vi "three string pad with zeroes.vi"(3 "String 3 input":string, 4 "String 2 input":string, 5 "String 1 input":string) -> (0 "String 3 output":string, 1 "String 2 output":string, 2 "String 1 output":string)   [LabVIEW 2017]
doc: "This takes two strings (presumably of 0s and 1s), and pads the shorter one with zeroes so that it has the same length as the longer one."
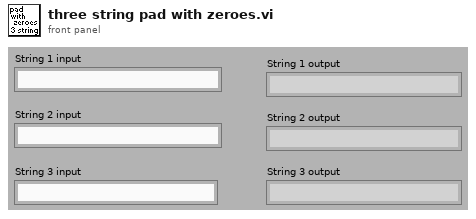
[diagram p1: front panel]
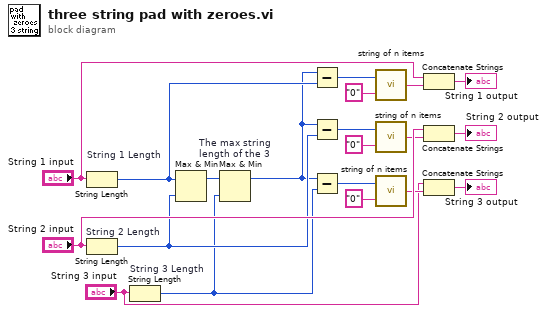
[diagram p0: block diagram]
diagram:
  n1 = String Length "String 1 Length"(string="String 1 input") -> (length=w9:i32)
  n2 = String Length "String 2 Length"(string="String 2 input") -> (length=w10:i32)
  n3 = String Length "String 3 Length"(string="String 3 input") -> (length=w1:i32)
  n4 = Max & Min(x=w9, y=w10) -> (max(x,y)=w8:i32)  [unwired: 1 out]
  n5 = Max & Min "The max string \nlength of the 3"(x=w8, y=w1) -> (max(x,y)=w2:i32)  [unwired: 1 out]
  n6 = Subtract(x=w2, y=w9) -> (x-y=w12:i32)
  n7 = Subtract(x=w2, y=w10) -> (x-y=w14:i32)
  n8 = Subtract(x=w2, y=w1) -> (x-y=w6:i32)
  n9 = call "string of n items.vi"("string"="0", "Numeric"=w12) -> ("String"=w15:string)
  n10 = call "string of n items.vi"("string"="0", "Numeric"=w14) -> ("String"=w16:string)
  n11 = call "string of n items.vi"("string"="0", "Numeric"=w6) -> ("String"=w5:string)
  n12 = Concatenate Strings("String 1 input", w15) -> (→"String 1 output":string)
  n13 = Concatenate Strings("String 2 input", w16) -> (→"String 2 output":string)
  n14 = Concatenate Strings("String 3 input", w5) -> (→"String 3 output":string)
